vi "CCC Server.vi"(8 "error in (no error)":errorcluster, 11 "Stop notifier":refnum<notifier>) -> (0 "error  out":errorcluster)   [LabVIEW 2010]
uses:
  NI_CCC.lvlib
panel:
  in  "port":u16=5555
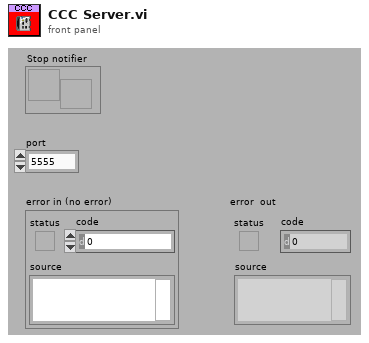
[diagram p1: front panel]
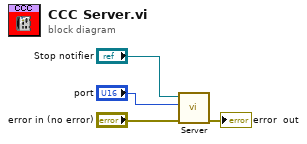
[diagram p0: block diagram]
diagram:
  n1 = call "Server.vi"("error in"="error in (no error)", "port (54444)"="port", "stop notifier"="Stop notifier") -> ("error  out"=→"error  out":errorcluster)  [unwired: 8 in]
